vi "publish data.vi"(6 "Self Enque? (False)":bool, 7 "Priority":enum16{"Normal", "High"}(ring), 8 "error in":errorcluster, 9 "data in":variant, 10 "command":string, 11 "refnum in":T1) -> (0 "error out":errorcluster, 3 "refnum in":T1)   [LabVIEW 2023, in "Publisher Subscriber.lvlib"]
uses:
  <userlib>/_Publisher Subscriber/Publisher Subscriber.lvlib
  <userlib>/_Publisher Subscriber/Controls/node refnum.ctl
  <userlib>/_Publisher Subscriber/Controls/node dvr data.ctl
  <userlib>/_Publisher Subscriber/Controls/data cluster.ctl
  <userlib>/_Publisher Subscriber/Controls/subscription bank ref.ctl
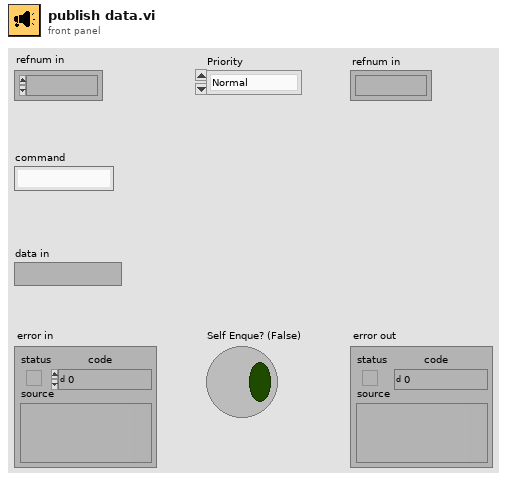
[diagram p1: front panel]
types:
  T1 = typedef "Publisher Subscriber.lvlib/node refnum.ctl" = refnum<vi>
  T2 = typedef "Publisher Subscriber.lvlib/data cluster.ctl" = cluster{"Command":string, "Data":variant}
  T3 = typedef "Publisher Subscriber.lvlib/node dvr data.ctl" = cluster{"queue ref":refnum<queue>, "Subscription Bank Ref":refnum<data-value>, "Command":string, "Data":variant, "Subscriptions []":set{string}, "Variables DVR Ref":refnum<data-value>}
  T4 = typedef "Publisher Subscriber.lvlib/subscription bank ref.ctl" = map{string, set{refnum<queue>}}
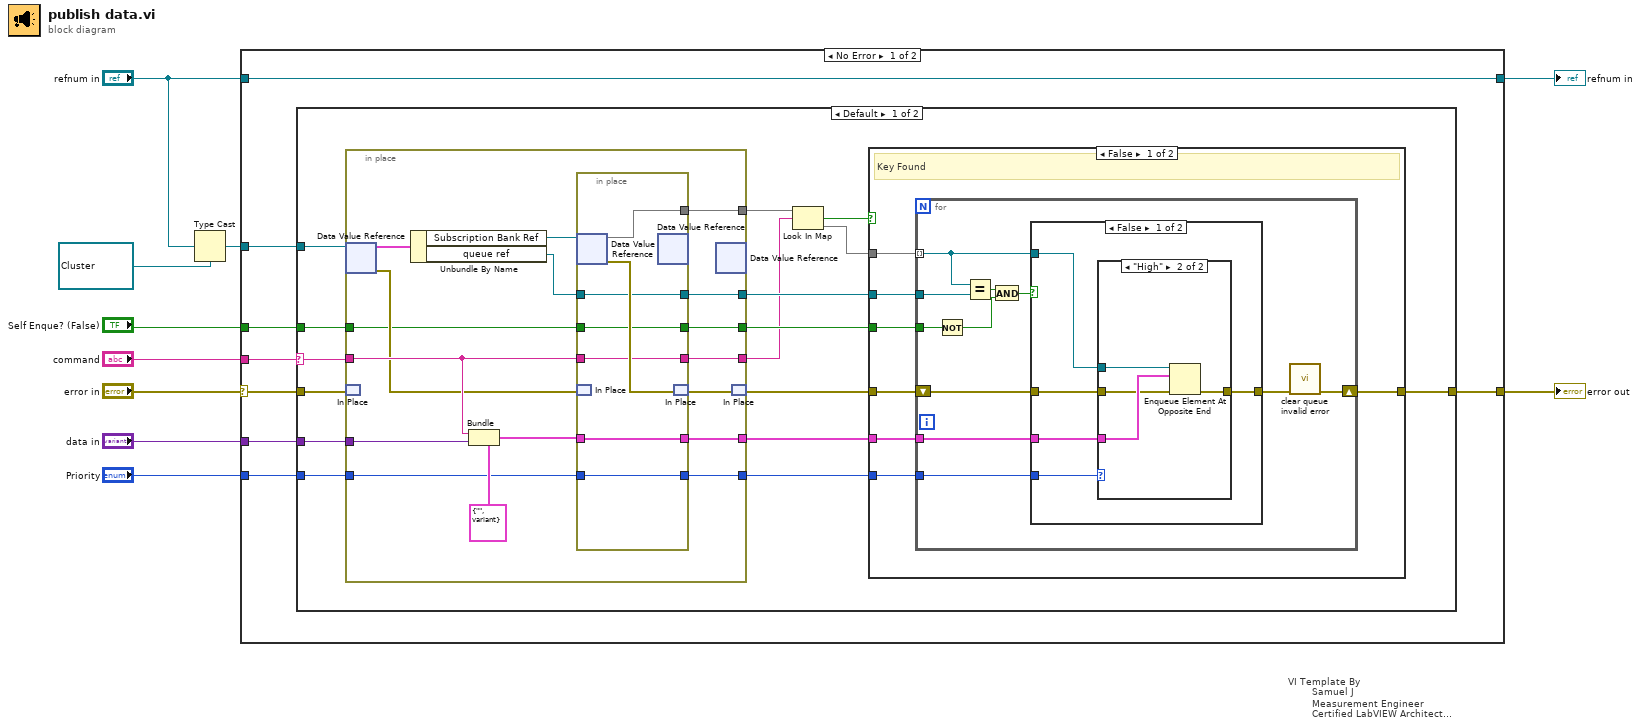
[diagram p0: block diagram]
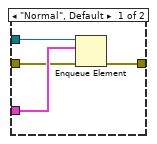
[diagram p2: hidden frame]
diagram:
  n1 = Type Cast(type=refnum<data-value> refnum ("data value reference"), x="refnum in") -> (*(type *) &x=w5:refnum<data-value>)
  n2 = case "VI Template By\n        Samuel J\n        Measurement Engineer\n        Certified LabVIEW Architect\n        Vestas Technology R&D Chennai" shown="No Error" "error in" {
    selector: "error in" -> [w18 w94]
    tunnel: [w11 w94] -> w9
    tunnel: "command" -> [w17 _]
    tunnel: "data in" -> [w16 _]
    tunnel: w5 -> [w15 _]
    tunnel: [w14 w93] -> w4
    tunnel: "refnum in" -> [w14 w93]
    tunnel: "Priority" -> [w13 _]
    tunnel: "Self Enque? (False)" -> [w12 _]
    frame No Error {
      n3 = case shown="Default" w17 {
        selector: w17 -> [w33 _]
        tunnel: w18 -> [w34 w92]
        tunnel: w16 -> [w32 _]
        tunnel: w15 -> [w31 _]
        tunnel: w13 -> [w30 _]
        tunnel: w12 -> [w29 _]
        tunnel: [w19 w92] -> w11
        frame Default {
          n4 = in-place {
            in-place-border: w33 -> [w81]
            in-place-border: w32 -> [w80]
            in-place-border: w30 -> [w76]
            in-place-border: w29 -> [w74]
            in-place-border: [w73] -> w26
            in-place-border: [w72] -> w25
            in-place-border: [w71] -> w24
            in-place-border: [w70] -> w23
            in-place-border: [w69] -> w21
            in-place-border: [w68] -> w20
            n5 = in-place-dvr #1(w31) -> (w84:T3, w77:errorcluster)
            n6 = in-place-match #2(w34) -> ()  [unwired: 1 out]
            n7 = Unbundle By Name(w84) -> ("Subscription Bank Ref"=w83:refnum<data-value>, "queue ref"=w75:refnum<queue>)
            n8 = Bundle(cluster=T2 {"Command"="", "Data"=variant} ("element"), "Command"=w81, "Data"=w80) -> (w79:T2)
            n9 = in-place {
              in-place-border: w81 -> [w87]
              in-place-border: w79 -> [w86]
              in-place-border: w76 -> [w85]
              in-place-border: w75 -> [w89]
              in-place-border: w74 -> [w88]
              in-place-border: [w90] -> w73
              in-place-border: [w89] -> w72
              in-place-border: [w88] -> w71
              in-place-border: [w87] -> w70
              in-place-border: [w86] -> w69
              in-place-border: [w85] -> w68
              n10 = in-place-dvr #3(w83) -> (w90:T4, w91:errorcluster)
              n11 = in-place-match #4(w77) -> ()  [unwired: 1 out]
              n12 = in-place-dvr #3() -> ()  [unwired: 1 in, 2 out]
              n13 = in-place-match #4(w91) -> (w78:errorcluster)
            }
            n14 = in-place-dvr #1() -> ()  [unwired: 1 in, 2 out]
            n15 = in-place-match #2(w78) -> (w22:errorcluster)
          }
          n16 = Look In Map(map=w26, key=w23) -> (key not found?=w28:bool, value=w27:set{refnum<queue>})  [unwired: 1 in]
          n17 = case shown="False" w28 {
            tunnel: w27 -> [w41 _]
            tunnel: w21 -> [w40 _]
            tunnel: [w39 w67] -> w19
            tunnel: w22 -> [w38 w67]
            tunnel: w20 -> [w37 _]
            tunnel: w25 -> [w36 _]
            tunnel: w24 -> [w35 _]
            frame False {
              # "Key Found"
              n18 = for {
                tunnel: w41 -> [w48] mode=indexing
                tunnel: w40 -> [w52]
                shift-right: [w42] -> w39
                shift-left: w38 -> [w51]
                tunnel: w37 -> [w50]
                tunnel: w36 -> [w49]
                tunnel: w35 -> [w47]
                n19 = Not(x=w47) -> (.not. x?=w44:bool)
                n20 = Equal?(x=w48, y=w49) -> (x = y?=w45:bool)
                n21 = And(x=w45, y=w44) -> (x .and. y?=w46:bool)
                n22 = case shown="False" w46 {
                  tunnel: w52 -> [w57 _]
                  tunnel: [w56 w66] -> w43
                  tunnel: w51 -> [w55 w66]
                  tunnel: w50 -> [w54 _]
                  tunnel: w48 -> [w53 _]
                  frame False {
                    n23 = case shown="\"High\"" w54 {
                      tunnel: w53 -> [w61 w65]
                      tunnel: w57 -> [w60 w64]
                      tunnel: [w59 w63] -> w56
                      tunnel: w55 -> [w58 w62]
                      frame "Normal", Default {
                        n24 = Enqueue Element(queue=w61, element=w60, error in (no error)=w58) -> (error out=w59:errorcluster)  [unwired: 1 in, 2 out]
                      }
                      frame "High" {
                        n25 = Enqueue Element At Opposite End(queue=w65, element=w64, error in (no error)=w62) -> (error out=w63:errorcluster)  [unwired: 1 in, 2 out]
                      }
                    }
                  }
                  frame True {
                  }
                }
                n26 = call <userlib>:"clear queue invalid error.vi"("error in (no error)"=w43) -> ("error in (no error)"=w42:errorcluster)  [unwired: 10 in]
              }
            }
            frame True {
              # "Key Not Found"
            }
          }
        }
        frame "" {
        }
      }
    }
    frame Error {
    }
  }
  "error out" <- w9
  "refnum in" <- w4
